vi "sync init semaphore.vi"(8 "error in (no error)":errorcluster, 11 "pointer in":u64) -> (0 "error out":errorcluster, 2 "Semaphore out":T1, 3 "offset pointer out":u64)   [LabVIEW 2013, in "Shared Memory runtime.lvclass"]
uses:
  Shared Memory runtime.lvclass
  <vilib>/NI/Pthreads for LabVIEW on Linux RT/Classes/Semaphore/Controls/reference.ctl
  <vilib>/NI/Pthreads for LabVIEW on Linux RT/Classes/Semaphore/Semaphore.lvclass
  <vilib>/NI/Pthreads for LabVIEW on Linux RT/Controls/Public/C Enums/pthread_process_shared.ctl
  <vilib>/NI/Pthreads for LabVIEW on Linux RT/POSIX Threads.lvlib
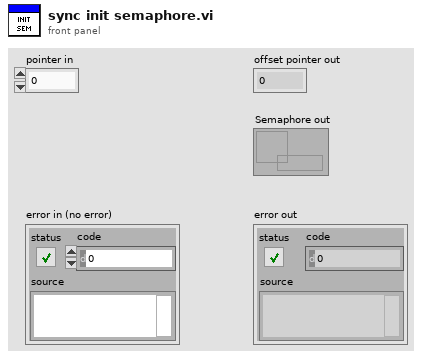
[diagram p1: front panel]
types:
  T1 = typedef "POSIX Threads.lvlib/Semaphore.lvclass/reference.ctl" = refnum<data-value>
  T2 = typedef "POSIX Threads.lvlib/pthread_process_shared.ctl" = enum16{"Private", "Shared"}
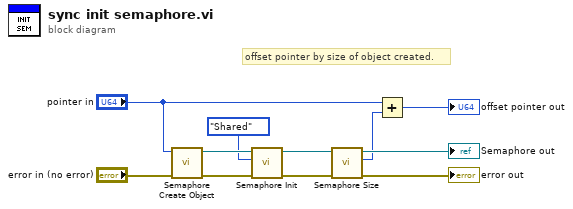
[diagram p0: block diagram]
diagram:
  # "offset pointer by size of object created."
  n1 = call <vilib>:"Semaphore Create Object.vi"("error in (no error)"="error in (no error)", "semaphore pointer"="pointer in") -> ("error out"=w8:errorcluster, "Semaphore out"=w9:T1)  [unwired: 8 in]
  n2 = call <vilib>:"Semaphore Init.vi"("error in (no error)"=w8, "process (private)"=pthread_process_shared."Shared", "Semaphore in"=w9) -> ("error out"=w5:errorcluster, "Semaphore out"=w6:T1)  [unwired: 7 in]
  n3 = call <vilib>:"Semaphore Size.vi"("error in (no error)"=w5, "Semaphore in"=w6) -> ("error out"=→"error out":errorcluster, "sem_t size (bytes)"=w2:u64, "Semaphore out"=→"Semaphore out":T1)  [unwired: 7 in]
  n4 = Add(x="pointer in", y=w2) -> (x+y=→"offset pointer out":u64)
